vi "read_stm.vi"() -> ()   [LabVIEW 2018]
uses:
  <vilib>/Instr/_visa.llb/VISA Configure Serial Port (Instr).vi
panel:
  in  "byte count":u32=1000
  in  "Enable Termination\nChar (T)":bool=TRUE
  out "size(s)":i32=501
  out "Waveform Chart":u8[](graph)
  out "length":i32=501
  out "return count":u32=501
  out "Numeric":i32=2311
  out "read buffer":string
  in  "stop":bool
  in  "Baud Rate":u32=115200
  in  "COM Port":refnum<visa-resource-name>="COM5"
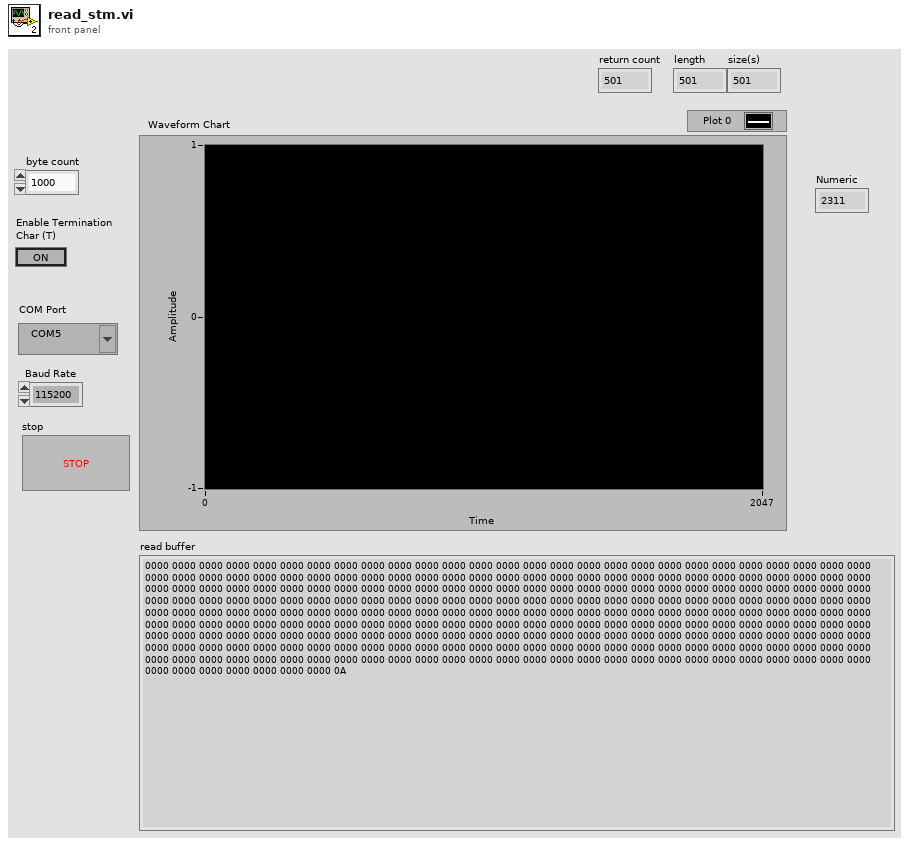
[diagram p1: front panel]
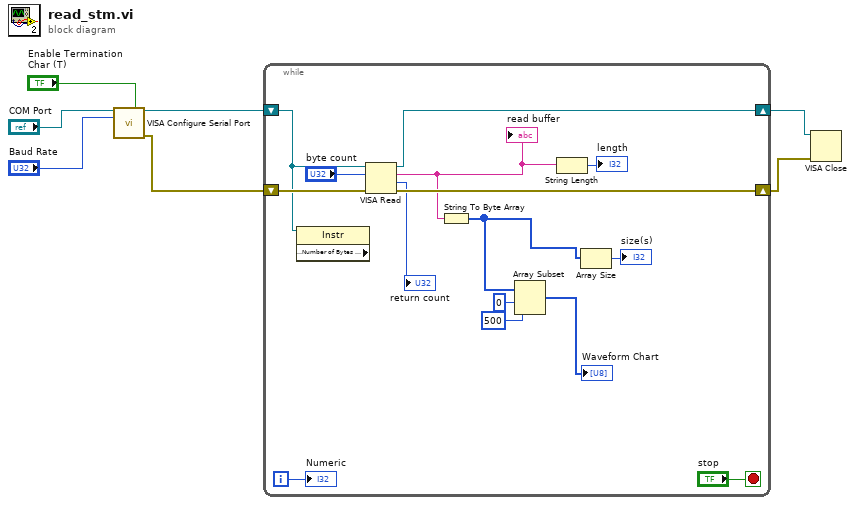
[diagram p0: block diagram]
diagram:
  n1 = call-poly "VISA Configure Serial Port"("VISA resource name"="COM Port", "Enable Termination\nChar (T)"="Enable Termination\nChar (T)", "baud rate (9600)"="Baud Rate") -> ("VISA resource name out"=w5:refnum<visa-resource-name>, "error out"=w4:errorcluster)  [unwired: 11 in]
  n2 = while {
    shift-right: [w15] -> w3
    shift-left: w5 -> [w14]
    shift-right: [w21] -> w2
    shift-left: w4 -> [w22]
    i -> [w19]
    stop <- "stop" stop-if-true
    n3 = property class="Instr" props=["Serial Settings:Number of Bytes at Serial Port"](reference=w14) -> ()  [unwired: 1 in, 3 out]
    n4 = VISA Read(VISA resource name=w14, byte count="byte count", error in (no error)=w22) -> (VISA resource name out=w15:refnum<visa-resource-name>, read buffer=w18:string, return count=→"return count":u32, error out=w21:errorcluster)
    "read buffer" <- w18
    n5 = String To Byte Array(string=w18) -> (unsigned byte array=w11:u8[])
    n6 = Array Subset(array=w11, index=0, length=500) -> (→"Waveform Chart":u8[])
    n7 = String Length(string=w18) -> (length=→"length":i32)
    n8 = Array Size(array=w11) -> (size(s)=→"size(s)":i32)
    "Numeric" <- w19
  }
  n9 = VISA Close(VISA resource name=w3, error in (no error)=w2) -> ()  [unwired: 1 out]
